vi "DPT Panel Voltage Panel Setup.vi"(5 "Channel List In":string, 7 "CDAQ?":bool=TRUE, 9 "Label List In":string[](array[string])) -> (6 "Channel List Out":string, 10 "Label List Out":string[](array[string]), 15 "Stream DC to File(out)?":bool)   [LabVIEW 2016]
uses:
  Type Definitions/DPT Channel Label.ctl
  Utility/Custom Pallet Controls/Custom Pallet String.ctl
  Utility/Custom Pallet Controls/Custom Pallet Forward.ctl
  Utility/Save File/File Setup (Public)/DPT Global Test Variables.vi
  Utility/Save File/File Setup.lvlib
panel:
  in  "Tab Control":enum32{"Page 1"}(tab)
  in  "Stream DC to File?":bool
  in  "DC Voltages":T1[](array[typedef])=[{"Label"="", "Record"=FALSE, "Index"=0, "Channel"=""}, {"Label"="", "Record"=FALSE, "Index"=0, "Channel"=""}, {"Label"="", "Record"=FALSE, "Index"=0, "Channel"=""}, {"Label"="", "Record"=FALSE, "Index"=0, "Channel"=""}, {"Label"="", "Record"=FALSE, "Index"=0, "Channel"=""}, {"Label"="", "Record"=FALSE, "Index"=0, "Channel"=""}, {"Label"="", "Record"=FALSE, "Index"=0, "Channel"=""}, {"Label"="", "Record"=FALSE, "Index"=0, "Channel"=""}]
  in  "stop":T3
  in  "AC Voltages":T1[](array[typedef])=[{"Label"="", "Record"=FALSE, "Index"=0, "Channel"=""}, {"Label"="", "Record"=FALSE, "Index"=0, "Channel"=""}, {"Label"="", "Record"=FALSE, "Index"=0, "Channel"=""}, {"Label"="", "Record"=FALSE, "Index"=0, "Channel"=""}, {"Label"="", "Record"=FALSE, "Index"=0, "Channel"=""}, {"Label"="", "Record"=FALSE, "Index"=0, "Channel"=""}, {"Label"="", "Record"=FALSE, "Index"=0, "Channel"=""}, {"Label"="", "Record"=FALSE, "Index"=0, "Channel"=""}]
  # "Note that the channels are hiddent in the \ncontrol typedef. so that the user cannot change them."
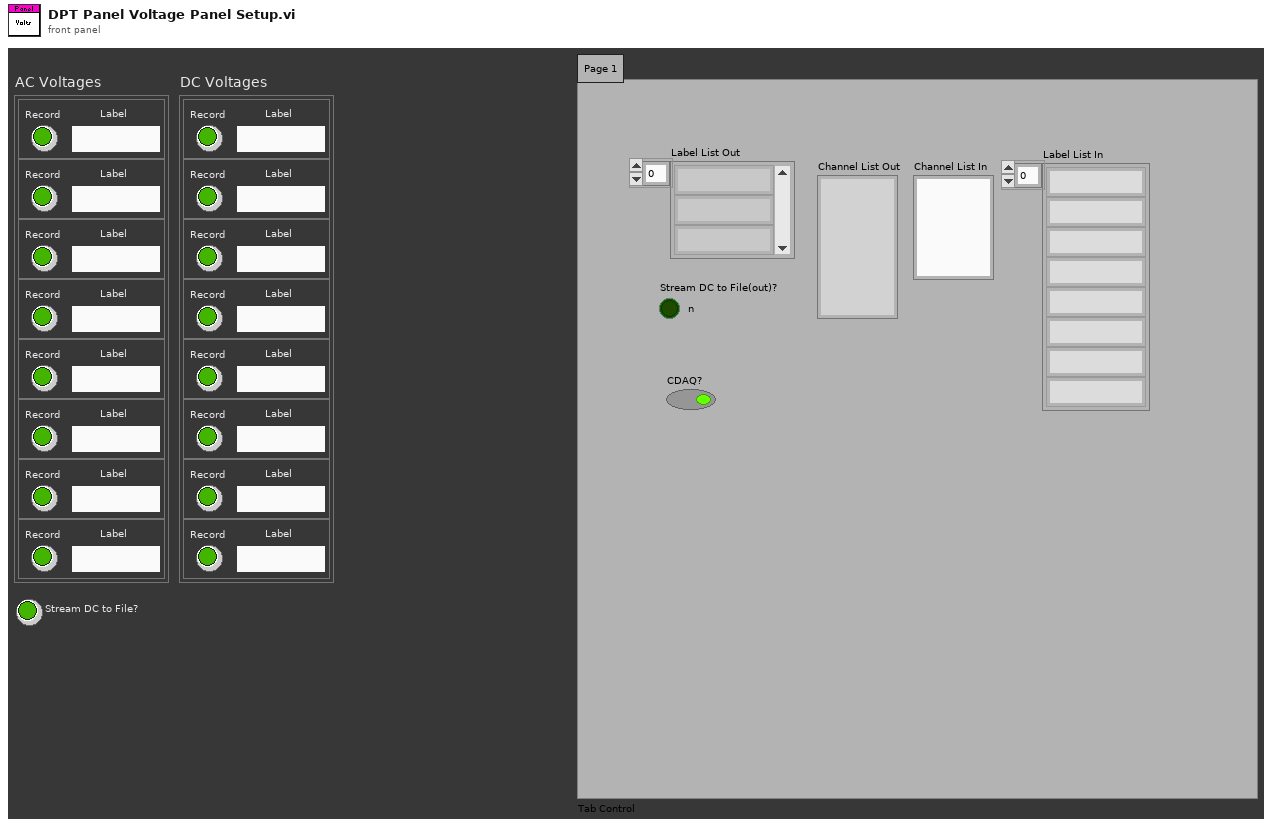
[diagram p1: front panel]
types:
  T1 = typedef "DPT Channel Label.ctl" = cluster{"Label":T2, "Record":bool, "Index":u32, "Channel":string}
  T2 = typedef "Custom Pallet String.ctl" = string
  T3 = typedef "Custom Pallet Forward.ctl" = bool
  T4 = typedef "File Setup.lvlib/DPT Global Type.ctl" = cluster{"Test Setup":cluster{"RH Resistor":dbl, "Temp Cal":dbl, "Temp Coeff":dbl, "Power On Threshold":dbl, "MA Filter Size":i32, "Weight Offset":dbl, "Temp Resistor":dbl, "Gas Enabled":bool, "Gas P. Resistor":dbl, "Scale Com":dbl, "W. Samps":i32, "Temp4mA Val":dbl, "Temp20mA Val":dbl, "RH4mA Val":dbl, "RH20mA Val":dbl, "GPres4mA Val":dbl, "Gpres20mA Val":dbl, "Smoothing":bool, "CDAQ":bool, "34970":bool, "34980":bool, "RH-IP":string, "RH-IP2":string, "RH-IP3":string, "CompVolume":dbl, "T45_Coeff.":dbl}, "Agilent Setup":cluster{"Scale Channel":string, "TC Channels":string, "VDC Discrete Channels":string, "RH Chan":string, "Temp Chan":string, "Tscale Channel":string, "RDB Channel":string, "Gas Temperature":string, "Gas Pressure":string, "Barometric Pressure":string, "Gas Feedback Chan":string}, "Directories":cluster{"Work File Directory":path, "Save File Directory":path, "Library Directory":path, "Data Backup Directory":path, "Data Backup Dir Fail":path, "Lab Directory":path}, "Test Information":cluster{"Model:":string, "Temperature:":string, "Engineer:":string, "Technician:":string, "Comments:":string, "Lab ID:":string, "TR Number:":string, "Test Number:":string, "Test Station:":string, "Empty Dryer Cold Weight:":dbl, "Serial Number:":string, "Build:":string, "Dryer Type":string, "Humidity":string, "Test Title per TR:":string}, "cDAQ Array Locations":cluster{"Scale Channel":string, "TC Channels":string, "VDC Discrete Channel":string, "RH Chan":string, "Temp Chan":string, "Tscale Channel":string, "RDB Channel":string, "Gas Temperature":string, "Gas Pressure":string, "Barometric Pressure":string, "Gas Feedback Chan":string}}
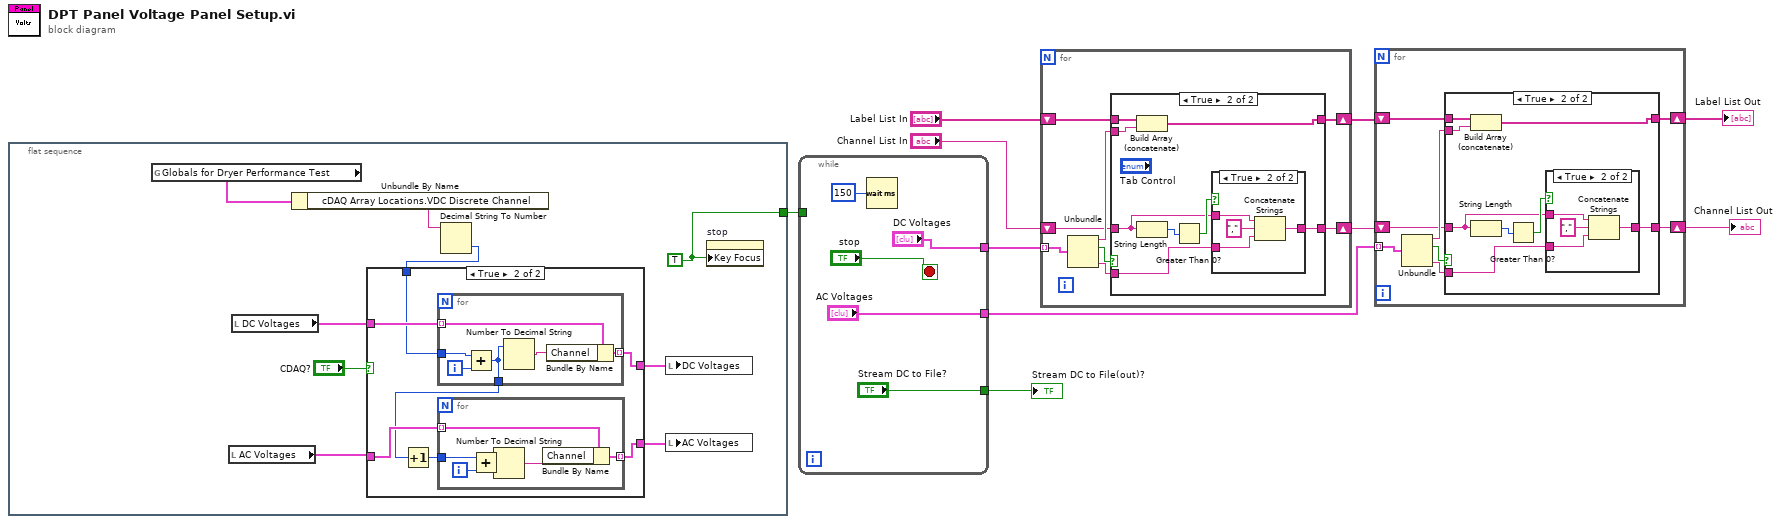
[diagram p0: block diagram]
diagram:
  n1 = flat-sequence {
    tunnel: [w19] -> w2
    frame #0 {
      w19 = TRUE ("Key Focus")
      n2 = global read "DPT Global Test Variables.vi" "Globals for Dryer Performance Test"() -> (w14:T4)
      n3 = local read "AC Voltages"() -> (w11:T1[])
      n4 = local read "DC Voltages"() -> (w12:T1[])
      n5 = Unbundle By Name(w14) -> ("cDAQ Array Locations.VDC Discrete Channel"=w15:string)
      n6 = Decimal String To Number(string=w15) -> (number=w13:i32)  [unwired: 2 in, 1 out]
      n7 = case shown="True" "CDAQ?" {
        tunnel: [w21 w26] -> w17
        tunnel: w12 -> [w21 w28]
        tunnel: [w20 w25] -> w16
        tunnel: w11 -> [w20 w24]
        tunnel: w13 -> [_ w27]
        frame False {
        }
        frame True {
          n8 = for {
            tunnel: w28 -> [w40] mode=indexing
            tunnel: w27 -> [w38]
            tunnel: [w36] -> w26 mode=indexing
            tunnel: [w35] -> w23
            i -> [w39]
            n9 = Add(x=w38, y=w39) -> (x+y=w35:i32)
            n10 = Number To Decimal String(number=w35) -> (decimal integer string=w37:string)  [unwired: 1 in]
            n11 = Bundle By Name(cluster=w40, "Channel"=w37) -> (w36:T1)
          }
          n12 = Increment(x=w23) -> (x+1=w22:i32)
          n13 = for {
            tunnel: w24 -> [w34] mode=indexing
            tunnel: w22 -> [w32]
            tunnel: [w29] -> w25 mode=indexing
            i -> [w33]
            n14 = Add(x=w32, y=w33) -> (x+y=w30:i32)
            n15 = Number To Decimal String(number=w30) -> (decimal integer string=w31:string)  [unwired: 1 in]
            n16 = Bundle By Name(cluster=w34, "Channel"=w31) -> (w29:T1)
          }
        }
      }
      n17 = local write "DC Voltages"(w17) -> ()
      n18 = local write "AC Voltages"(w16) -> ()
      n19 = property on="stop" class="Bool"("Key Focus"=w19) -> ()  [unwired: 2 in, 2 out]
    }
  }
  n20 = while {
    tunnel: ["DC Voltages"] -> w10
    tunnel: ["AC Voltages"] -> w5
    tunnel: w2 -> [_]
    tunnel: ["Stream DC to File?"] -> w1
    stop <- "stop" stop-if-true
    n21 = Wait (ms)(milliseconds to wait=u32 150) -> ()  [unwired: 1 out]
  }
  "Stream DC to File(out)?" <- w1
  n22 = for {
    tunnel: w10 -> [w53] mode=indexing
    shift-right: [w50] -> w7
    shift-left: "Label List In" -> [w51]
    shift-right: [w49] -> w6
    shift-left: "Channel List In" -> [w48]
    n23 = Unbundle(w53) -> ("Label"=w52:T2, "Record"=w46:bool, "Channel"=w47:string)  [unwired: 1 out]
    n24 = case shown="True" w46 {
      tunnel: w52 -> [_ w63]
      tunnel: w51 -> [w55 w62]
      tunnel: [w55 w61] -> w50
      tunnel: w48 -> [w54 w58]
      tunnel: [w54 w57] -> w49
      tunnel: w47 -> [_ w56]
      frame False {
      }
      frame True {
        n25 = Build Array (concatenate)(w62, w63) -> (w61:T2[])
        n26 = String Length(string=w58) -> (length=w60:i32)
        n27 = Greater Than 0?(x=w60) -> (x > 0?=w59:bool)
        n28 = case shown="True" w59 {
          tunnel: w58 -> [_ w68]
          tunnel: w56 -> [w64 w66]
          tunnel: [w64 w65] -> w57
          frame False {
          }
          frame True {
            n29 = Concatenate Strings(w68, "," ("string"), w66) -> (w65:string)
          }
        }
      }
    }
  }
  n30 = for {
    tunnel: w5 -> [w76] mode=indexing
    shift-right: [w73] -> w4
    shift-left: w7 -> [w74]
    shift-right: [w72] -> w3
    shift-left: w6 -> [w71]
    n31 = Unbundle(w76) -> ("Label"=w75:T2, "Record"=w69:bool, "Channel"=w70:string)  [unwired: 1 out]
    n32 = case shown="True" w69 {
      tunnel: w75 -> [_ w86]
      tunnel: w74 -> [w78 w85]
      tunnel: [w78 w84] -> w73
      tunnel: w71 -> [w77 w81]
      tunnel: [w77 w80] -> w72
      tunnel: w70 -> [_ w79]
      frame False {
      }
      frame True {
        n33 = Build Array (concatenate)(w85, w86) -> (w84:T2[])
        n34 = String Length(string=w81) -> (length=w83:i32)
        n35 = Greater Than 0?(x=w83) -> (x > 0?=w82:bool)
        n36 = case shown="True" w82 {
          tunnel: w81 -> [_ w91]
          tunnel: w79 -> [w87 w89]
          tunnel: [w87 w88] -> w80
          frame False {
          }
          frame True {
            n37 = Concatenate Strings(w91, "," ("string"), w89) -> (w88:string)
          }
        }
      }
    }
  }
  "Label List Out" <- w4
  "Channel List Out" <- w3
